vi "input.vi"(8 "error in":errorcluster, 10 "input allocation":T1, 11 "DAQmx Watchdog runtime in":refnum<class "DAQmx Watchdog runtime.lvclass">) -> (0 "error out":errorcluster, 2 "input data":T1, 3 "DAQmx Watchdog runtime out":refnum<class "DAQmx Watchdog runtime.lvclass">)   [LabVIEW 2014, in "DAQmx Watchdog runtime.lvclass"]
doc: "Provides an interface for reading data from a module at runtime. While this interface performs no operations, a child should provide an override which may read from any open sessions, references, or interfaces."
uses:
  DAQmx Watchdog runtime.lvclass
  <vilib>/NI/Tag Bus/table/data table.ctl
  input user data.ctl
  DAQmx Watchdog runtime.lvclass/DAQmx Watchdog runtime.ctl
  <resource>/objmgr/daqmx.rc
  <vilib>/NI/Tag Bus/table/data table.lvlib
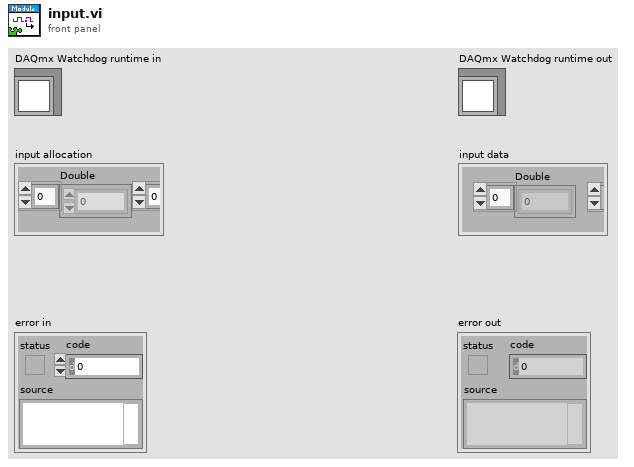
[diagram p1: front panel]
types:
  T1 = typedef "tag bus.lvlib/data table.lvlib/data table.ctl" = cluster{"Double":dbl[], "Single":sgl[], "I64":i64[], "I32":i32[], "I16":i16[], "I8":i8[], "U64":u64[], "U32":u32[], "U16":u16[], "U8":u8[], "Boolean":bool[], "String":string[], "Array of Double":cluster{"DBL Array":dbl[]}[], "Array of Single":cluster{"SGL Array":sgl[]}[], "Array of I64":cluster{"I64 Array":i64[]}[], "Array of I32":cluster{"I32 Array":i32[]}[], "Array of I16":cluster{"I16 Array":i16[]}[], "Array of I8":cluster{"I8 Array":i8[]}[], "Array of U64":cluster{"U64 Array":u64[]}[], "Array of U32":cluster{"U32 Array":u32[]}[], "Array of U16":cluster{"U16 Array":u16[]}[], "Array of U8":cluster{"U8 Array":u8[]}[], "Array of Boolean":cluster{"Boolean Array":bool[]}[], "Array of String":cluster{"String Array":string[]}[]}
  T2 = typedef "DAQmx Watchdog runtime.lvclass/input user data.ctl" = cluster{"Watchdog Expired":bool}
  T3 = typedef "DAQmx Watchdog configuration.lvclass/input data indices.ctl" = cluster{"Boolean.Watchdog Expired":i32}
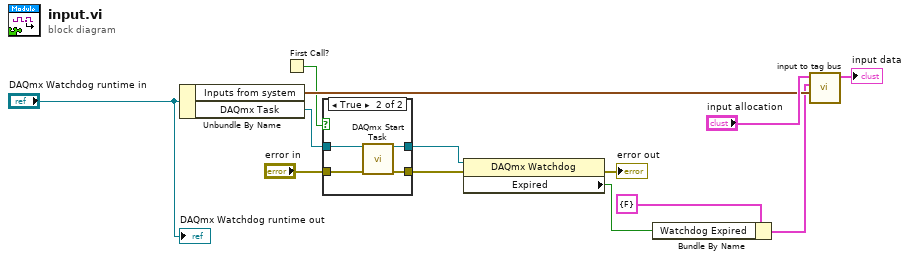
[diagram p0: block diagram]
diagram:
  n1 = Unbundle By Name("DAQmx Watchdog runtime in") -> ("Inputs from system"=w10:T3, "DAQmx Task"=w4:refnum<k21>)
  n2 = First Call?() -> (First Call?: T/F=w5:bool)
  n3 = case shown="True" w5 {
    tunnel: w4 -> [w14 w19]
    tunnel: "error in" -> [w15 w18]
    tunnel: [w15 w17] -> w2
    tunnel: [w14 w16] -> w1
    frame False {
    }
    frame True {
      n4 = call <vilib>:"DAQmx Start Task.vi"("task/channels in"=w19, "error in"=w18) -> ("task out"=w16:refnum<k21>, "error out"=w17:errorcluster)  [unwired: 12 in]
    }
  }
  n5 = property class="DAQmx Watchdog"(reference=w1, error in=w2) -> (error out=→"error out":errorcluster, "Expired"=w8:bool)  [unwired: 1 out]
  n6 = Bundle By Name(cluster=T2 {"Watchdog Expired"=FALSE} ("data cluster"), "Watchdog Expired"=w8) -> (w6:T2)
  n7 = call "input to tag bus.vi"("indices"=w10, "data cluster"=w6, "tag bus in"="input allocation") -> ("tag bus out"=→"input data":T1)  [unwired: 8 in]
  "DAQmx Watchdog runtime out" <- "DAQmx Watchdog runtime in"
